vi "get index definition.vi"(10 "channel classification":T1, 11 "fixed channel configuration in":refnum<class "fixed channel configuration.lvclass">) -> (1 "valid?":bool, 2 "index cluster":variant, 3 "fixed channel configuration out":refnum<class "fixed channel configuration.lvclass">)   [LabVIEW 2013, in "fixed channel configuration.lvclass"]
uses:
  fixed channel configuration.lvclass
  <vilib>/NI/Tag Bus Module Framework/channel/channel classification.ctl
  <vilib>/Utility/VariantDataType/VariantType.lvlib
  <vilib>/NI/Tag Bus Module Framework/channel/TBM channel.lvclass
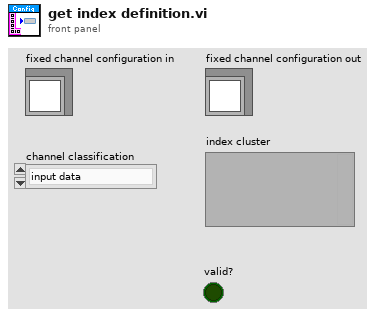
[diagram p1: front panel]
types:
  T1 = typedef "TBM channel.lvclass/channel classification.ctl" = enum16{"input data", "output data", "processing parameter", "processing result"}
  T2 = typedef "fixed channel configuration.lvclass/index type definitions.ctl" = cluster{"input indices":variant, "parameter indices":variant, "result indices":variant, "output indices":variant}
  T3 = typedef "VariantType.lvlib/Type.ctl" = enum8{"Invalid Type", "Void", "I8", "I16", "I32", "I64", "U8", "U16", "U32", "U64", "Single Float", "Double Float", "Extended Float", "Single Complex", "Double Complex", "Extended Complex", "Enum U8", "Enum U16", "Enum U32", "Enum U64", "Single Float With Unit", "Double Float With Unit", "Extended Float With Unit", "Single Complex with Unit", "Double Complex with Unit", "Extended Complex with Unit", "Boolean", "String", "Path", "Picture", "Tag", "Array", "Cluster", "Variant", "LV Variant", "Waveform", "Timestamp", "Digital Waveform", "Digital Data", "ExpressData", "Refnum", "External Data", "VI", "Poly VI", "LabVIEW Class Instance", "Fixed Point"}
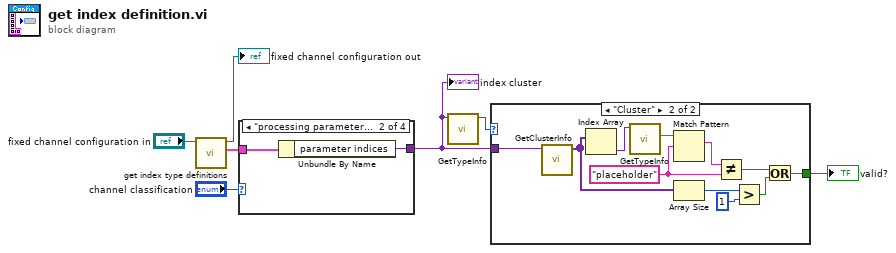
[diagram p0: block diagram]
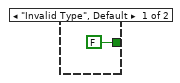
[diagram p2: hidden frame]
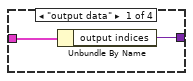
[diagram p3: hidden frame]
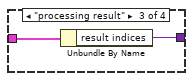
[diagram p4: hidden frame]
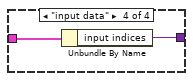
[diagram p5: hidden frame]
diagram:
  n1 = call-dynamic "get index type definitions.vi"("fixed channel configuration in"="fixed channel configuration in") -> ("index type defs"=w3:T2, "fixed channel configuration out"=→"fixed channel configuration out":refnum<class "fixed channel configuration.lvclass">)  [unwired: 9 in]
  n2 = case shown="\"processing parameter\"" "channel classification" {
    tunnel: w3 -> [w9 w11 w13 w15]
    tunnel: [w8 w10 w12 w14] -> w2
    frame "output data" {
      n3 = Unbundle By Name(w9) -> ("output indices"=w8:variant)
    }
    frame "processing parameter" {
      n4 = Unbundle By Name(w11) -> ("parameter indices"=w10:variant)
    }
    frame "processing result" {
      n5 = Unbundle By Name(w13) -> ("result indices"=w12:variant)
    }
    frame "input data" {
      n6 = Unbundle By Name(w15) -> ("input indices"=w14:variant)
    }
  }
  "index cluster" <- w2
  n7 = call <vilib>:"GetTypeInfo.vi"("Variant"=w2) -> ("Type Enum"=w5:T3)  [unwired: 6 in, 4 out]
  n8 = case shown="\"Cluster\"" w5 {
    tunnel: [FALSE w17] -> w1
    tunnel: w2 -> [_ w27]
    frame "Invalid Type", Default {
    }
    frame "Cluster" {
      w20 = "placeholder" ("regular expression")
      n9 = call <vilib>:"GetClusterInfo.vi"("Variant"=w27) -> ("Cluster Elements"=w24:variant[])  [unwired: 9 in, 1 out]
      n10 = Index Array(array=w24) -> (element=w23:variant)  [unwired: 1 in]
      n11 = call <vilib>:"GetTypeInfo.vi"("Variant"=w23) -> ("Name"=w22:string)  [unwired: 6 in, 4 out]
      n12 = Match Pattern(string=w22, regular expression=w20) -> (match substring=w21:string)  [unwired: 1 in, 3 out]
      n13 = Array Size(array=w24) -> (size(s)=w26:i32)
      n14 = Not Equal?(x=w21, y=w20) -> (x != y?=w19:bool)
      n15 = Greater?(x=w26, y=1) -> (0:w18:bool)
      n16 = Or(x=w19, y=w18) -> (x .or. y?=w17:bool)
    }
  }
  "valid?" <- w1
